vi "error - braces missing.vi"(8 "error in (no error)":errorcluster) -> (0 "error out":errorcluster)   [LabVIEW 2024, in "controls manager.lvlib"]
uses:
  controls manager.lvlib
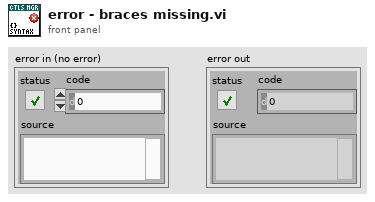
[diagram p1: front panel]
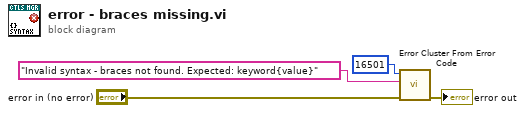
[diagram p0: block diagram]
diagram:
  n1 = call <vilib>:"Error Cluster From Error Code.vi"("error in (no error)"="error in (no error)", "error message (\"\")"="Invalid syntax - braces not found. Expected: keyword{value}", "error code (0)"=16501) -> ("error out"=→"error out":errorcluster)  [unwired: 6 in]
